vi "Combined Steering and Drive Control Test.vi"() -> ()   [LabVIEW 2009]
uses:
  Motor Encoder Global.vi
  Motor Output Global.vi
  Inner Control/Drive Control Global DO NOT MODIFY!.vi
panel:
  in  "Steering Position Offset":i32
  out "Drive Encoder":i32
  out "Drive Encoder tick/count":i32
  out "Drive Encoder ft/sec":fxp<+/-,14,4>
  in  "Drive Enable":bool
  in  "Drive Speed Set Point (ft/sec)":fxp<+/-,14,4>
  in  "Drive Speed Control Feedback Gain":fxp<+/-,20,5>
  in  "Manual Override?":bool
  in  "Steering Position Target":i32
  in  "Steering Enable":bool
  in  "Steering Proportional Control Feedback Gain":fxp<+/-,20,5>
  in  "stop":bool
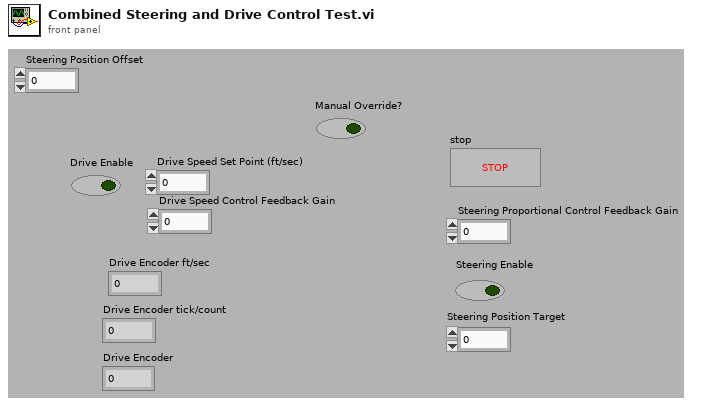
[diagram p1: front panel]
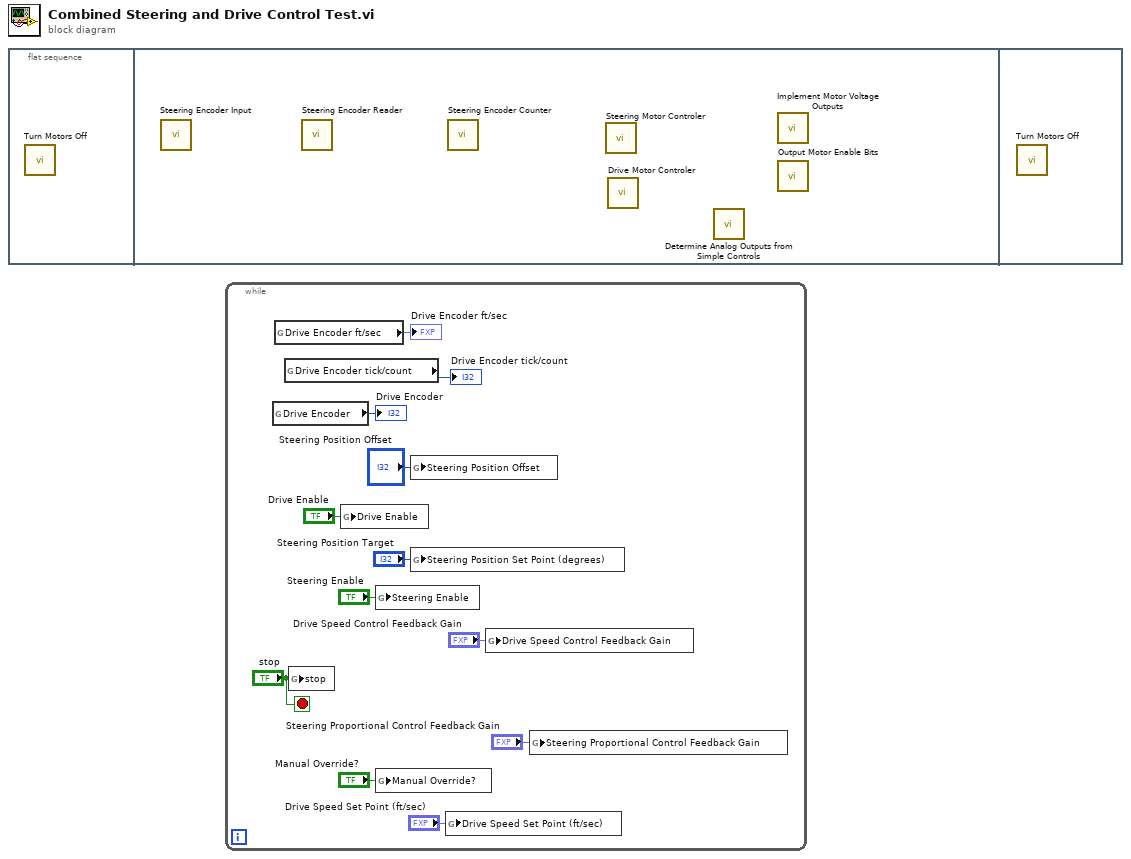
[diagram p0: block diagram]
diagram:
  n1 = flat-sequence {
    frame #0 {
      n2 = call "Turn Motors Off.vi"() -> ()  [unwired: 1 in]
    }
    frame #1 {
      n3 = call "Steering Encoder Input.vi"() -> ()  [unwired: 1 in]
      n4 = call "Steering Encoder Reader.vi"() -> ()  [unwired: 1 in]
      n5 = call "Steering Encoder Counter.vi"() -> ()  [unwired: 1 in]
      n6 = call "Steering Motor Controler.vi"() -> ()  [unwired: 1 in]
      n7 = call "Drive Motor Controler.vi"() -> ()  [unwired: 1 in]
      n8 = call "Determine Analog Outputs from Simple Controls.vi"() -> ()  [unwired: 1 in]
      n9 = call "Implement Motor Voltage Outputs.vi"() -> ()  [unwired: 1 in]
      n10 = call "Output Motor Enable Bits.vi"() -> ()  [unwired: 1 in]
    }
    frame #2 {
      n11 = call "Turn Motors Off.vi"() -> ()  [unwired: 1 in]
    }
  }
  n12 = while {
    stop <- "stop" stop-if-true
    n13 = global read "Motor Encoder Global.vi" "Drive Encoder"() -> (→"Drive Encoder":i32)
    n14 = global read "Drive Control Global DO NOT MODIFY!.vi" "Drive Encoder ft/sec"() -> (→"Drive Encoder ft/sec":fxp<+/-,18,8>)
    n15 = global read "Drive Control Global DO NOT MODIFY!.vi" "Drive Encoder tick/count"() -> (→"Drive Encoder tick/count":u32)
    n16 = global write "Motor Encoder Global.vi" "stop"("stop") -> ()
    n17 = global write "Motor Output Global.vi" "Drive Enable"("Drive Enable") -> ()
    n18 = global write "Motor Output Global.vi" "Steering Enable"("Steering Enable") -> ()
    n19 = global write "Motor Output Global.vi" "Manual Override?"("Manual Override?") -> ()
    n20 = global write "Motor Encoder Global.vi" "Steering Position Offset"("Steering Position Offset") -> ()
    n21 = global write "Motor Encoder Global.vi" "Steering Position Set Point (degrees)"("Steering Position Target") -> ()
    n22 = global write "Motor Encoder Global.vi" "Drive Speed Set Point (ft/sec)"("Drive Speed Set Point (ft/sec)") -> ()
    n23 = global write "Motor Encoder Global.vi" "Drive Speed Control Feedback Gain"("Drive Speed Control Feedback Gain") -> ()
    n24 = global write "Motor Encoder Global.vi" "Steering Proportional Control Feedback Gain"("Steering Proportional Control Feedback Gain") -> ()
  }
